vi "TBM.SetPos.vi"(7 "Caller Control Refnum":refnum<vi>, 8 "error in (no error)":errorcluster, 10 "Position":T2, 11 "Menu VI":refnum<vi>) -> (0 "error out":errorcluster, 1 "Ctrl Screen Bounds":T1, 2 "FP Screen Bounds":T1, 3 "Menu VI":refnum<vi>)   [LabVIEW 2013, in "ToolbarMenu.lvlib"]
uses:
  ToolbarMenu.lvlib
  MenuPosition.ctl
  <vilib>/Utility/miscctls.llb/LVRectTypeDef.ctl
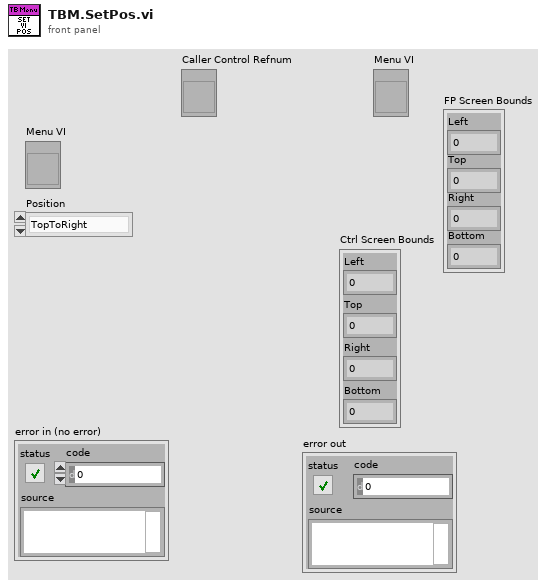
[diagram p1: front panel]
types:
  T1 = typedef "LVRectTypeDef.ctl" = cluster{"Left":i16, "Top":i16, "Right":i16, "Bottom":i16}
  T2 = typedef "ToolbarMenu.lvlib/MenuPosition.ctl" = enum16{"TopToRight", "BottomToRight", "TopToLeft", "BottomToLeft"}
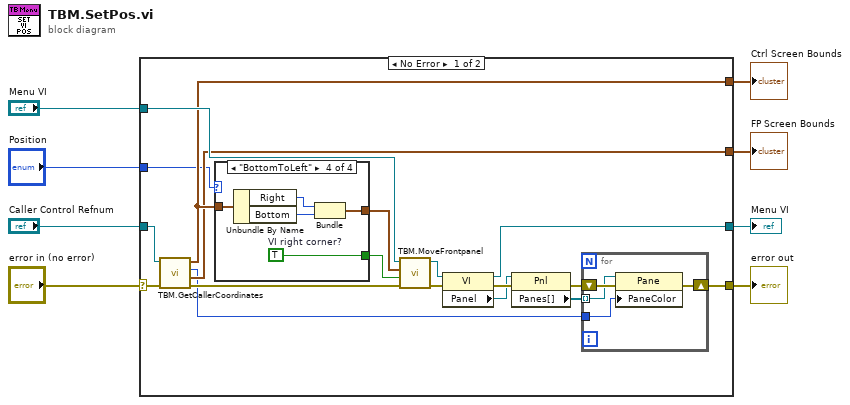
[diagram p0: block diagram]
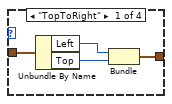
[diagram p2: hidden frame]
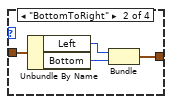
[diagram p3: hidden frame]
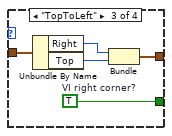
[diagram p4: hidden frame]
diagram:
  n1 = case shown="No Error" "error in (no error)" {
    selector: "error in (no error)" -> [w22 w50]
    tunnel: [w10 w49] -> w8
    tunnel: "Menu VI" -> [w26 w49]
    tunnel: [w11 w50] -> w3
    tunnel: "Caller Control Refnum" -> [w24 _]
    tunnel: "Position" -> [w18 _]
    tunnel: [w20 _] -> w2
    tunnel: [w19 _] -> w1
    frame No Error {
      n2 = call "TBM.GetCallerCoordinates.vi"("error in (no error)"=w22, "Control in"=w24) -> ("error out"=w23:errorcluster, "FP Screen Bounds"=w19:T1, "Pane Color"=w13:u32, "Ctrl Screen Bounds"=w20:T1)  [unwired: 6 in]
      n3 = case shown="\"BottomToLeft\"" w18 {
        tunnel: [_ _ w43 w48] -> w25
        tunnel: w20 -> [w32 w36 w40 w45]
        tunnel: [w31 w35 w39 w44] -> w21
        frame "TopToRight" {
          n4 = Unbundle By Name(w32) -> ("Left"=w34:i16, "Top"=w33:i16)
          n5 = Bundle("Left"=w34, "Top"=w33) -> (w31:cluster{"Left":i16, "Top":i16})  [unwired: 1 in]
        }
        frame "BottomToRight" {
          n6 = Unbundle By Name(w36) -> ("Left"=w38:i16, "Bottom"=w37:i16)
          n7 = Bundle("Left"=w38, "Bottom"=w37) -> (w35:cluster{"Left":i16, "Bottom":i16})  [unwired: 1 in]
        }
        frame "TopToLeft" {
          w43 = TRUE  # VI right corner?
          n8 = Unbundle By Name(w40) -> ("Right"=w42:i16, "Top"=w41:i16)
          n9 = Bundle("Right"=w42, "Top"=w41) -> (w39:cluster{"Right":i16, "Top":i16})  [unwired: 1 in]
        }
        frame "BottomToLeft" {
          w48 = TRUE  # VI right corner?
          n10 = Unbundle By Name(w45) -> ("Right"=w47:i16, "Bottom"=w46:i16)
          n11 = Bundle("Right"=w47, "Bottom"=w46) -> (w44:cluster{"Right":i16, "Bottom":i16})  [unwired: 1 in]
        }
      }
      n12 = call "TBM.MoveFrontpanel.vi"("error in (no error)"=w23, "VI right corner?"=w25, "Screen Position"=w21, "VI in"=w26) -> ("error out"=w12:errorcluster, "VI out"=w15:refnum<vi>)  [unwired: 6 in]
      n13 = property class="VI"(reference=w15, error in=w12) -> (reference out=w10:refnum<vi>, error out=w17:errorcluster, "Panel"=w16:refnum<vi>)
      n14 = property class="Pnl"(reference=w16, error in=w17) -> (error out=w9:errorcluster, "Panes[]"=w14:refnum<vi>[])  [unwired: 1 out]
      n15 = for {
        shift-right: [w29] -> w11
        shift-left: w9 -> [w30]
        tunnel: w14 -> [w28] mode=indexing
        tunnel: w13 -> [w27]
        n16 = property class="Pane"(reference=w28, error in=w30, "PaneColor"=w27) -> (error out=w29:errorcluster)  [unwired: 1 out]
      }
    }
    frame Error {
    }
  }
  "Menu VI" <- w8
  "error out" <- w3
  "Ctrl Screen Bounds" <- w2
  "FP Screen Bounds" <- w1
